vi "Linear Ramp [U16].vi"(0 "Increment (1)":u16=1, 3 "# Elements":i32, 4 "Start (0)":u16) -> (5 "Ramp":u16[](array[numeric]))   [LabVIEW 2021, in "Arrays.lvlib"]
uses:
  Arrays.lvlib
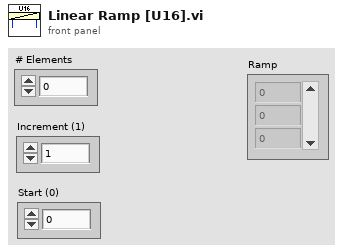
[diagram p1: front panel]
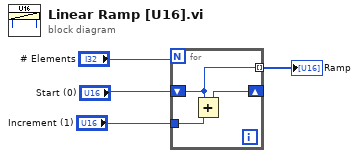
[diagram p0: block diagram]
diagram:
  n1 = for {
    N: "# Elements" -> [_]
    shift-right: [w6] -> _
    shift-left: "Start (0)" -> [w5]
    tunnel: "Increment (1)" -> [w7]
    tunnel: [w5] -> w1 mode=indexing
    n2 = Add(x=w5, y=w7) -> (x+y=w6:u16)
  }
  "Ramp" <- w1
